vi "Motion_Convert Loader Move Data.vi"(5 "Loader Move Data":T1 {"Connect Velocity" format="%_7g"; "Loader Velocity" format="%_7g"; "Load Position" format="%_7g"; "Connect Position" format="%_7g"; "Loader Accel/Decel" format="%_7g"}) -> (6 "Loader Move Register Data":u16[](array[numeric]))   [LabVIEW 2010]
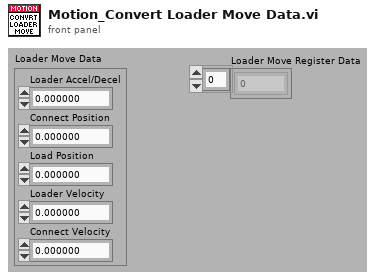
[diagram p1: front panel]
types:
  T1 = cluster{"Loader Accel/Decel":dbl, "Connect Position":dbl, "Load Position":dbl, "Loader Velocity":dbl, "Connect Velocity":dbl}
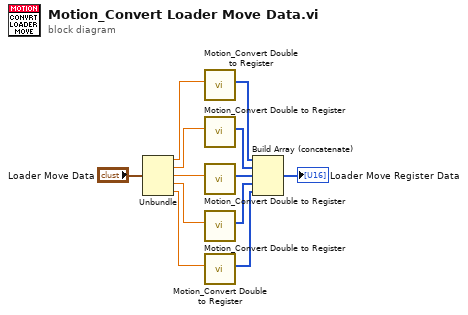
[diagram p0: block diagram]
diagram:
  n1 = Unbundle("Loader Move Data") -> ("Loader Accel/Decel"=w6:dbl, "Connect Position"=w5:dbl, "Load Position"=w3:dbl, "Loader Velocity"=w4:dbl, "Connect Velocity"=w2:dbl)
  n2 = call "Motion_Convert Double to Register.vi"("Double Value"=w6) -> ("U16 Array"=w12:u16[])  [unwired: 10 in]
  n3 = call "Motion_Convert Double to Register.vi"("Double Value"=w5) -> ("U16 Array"=w11:u16[])  [unwired: 10 in]
  n4 = call "Motion_Convert Double to Register.vi"("Double Value"=w3) -> ("U16 Array"=w10:u16[])  [unwired: 10 in]
  n5 = call "Motion_Convert Double to Register.vi"("Double Value"=w4) -> ("U16 Array"=w9:u16[])  [unwired: 10 in]
  n6 = call "Motion_Convert Double to Register.vi"("Double Value"=w2) -> ("U16 Array"=w1:u16[])  [unwired: 10 in]
  n7 = Build Array (concatenate)(w12, w11, w10, w9, w1) -> (→"Loader Move Register Data":u16[])
